vi "saturated boiling temp.vi"(8 "error in (no error)":errorcluster, 11 "pPa":dbl) -> (0 "error out":errorcluster, 3 "function return":dbl)   [LabVIEW 2011, in "fsteam.lvlib"]
doc: "extern double saturated_boiling_temp(double pPa);"
uses:
  <userlib>/fsteam/fsteam.lvlib
  <userlib>/fsteam/fsteam.dll
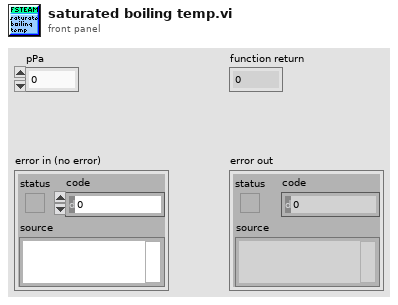
[diagram p1: front panel]
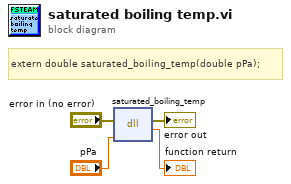
[diagram p0: block diagram]
diagram:
  # "extern double saturated_boiling_temp(double pPa);"
  n1 = dll-call lib="C:/Program Files (x86)/National Instruments/LabVIEW 2011/user.lib/fsteam/fsteam.*" fn="saturated_boiling_temp"(error in="error in (no error)", "pPa"="pPa") -> (error out=→"error out":errorcluster, →"function return":dbl)  [unwired: 3 in, 1 out]
